vi "PWM Driver.vi"(5 "PWM Configuration (\"\")":string, 6 "Drv Refnum":T1, 7 "PWM Command":T2=enum."MEASURE", 8 "error in (no error)":errorcluster, 10 "PWM Stimulus":T4={"Zero"=FALSE, "Blank Screen"=FALSE, "Offset"=FALSE, "Offset Value"=4.0, "Frequency (MHz)"=0.0}) -> (0 "error out":errorcluster, 1 "Variant Output":string, 2 "PWM Measurement":T3 caption="This reading is always in the base units\ni.e. V, A, Ohms, Hz, Sec, etc." format="%#_10f", 4 "dup Drv Refnum":T1)   [LabVIEW 2011]
uses:
  PWM Measurement.ctl
  PWM Parameters.ctl
  PWM Command.ctl
  PWM Driver Ref.ctl
panel:
  in  "DEBUG?":bool
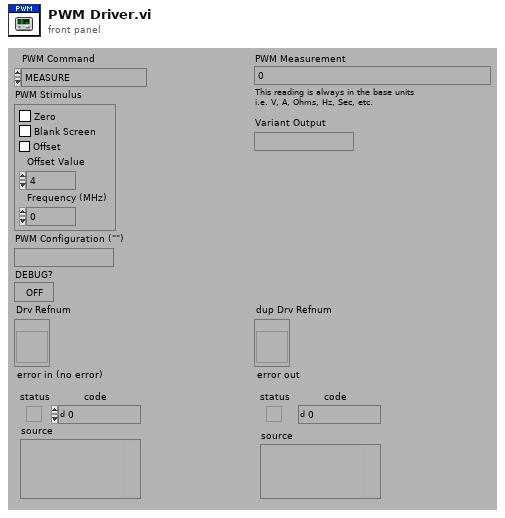
[diagram p1: front panel]
types:
  T1 = typedef "PWM Driver Ref.ctl" = refnum<vi>
  T2 = typedef "PWM Command.ctl" = enum16{"LOAD", "INITIALIZE", "PRESET", "GET STIMULUS", "SET STIMULUS", "MEASURE", "RELEASE", "UNLOAD", "GET CALIBRATION", "CALIBRATE"}
  T3 = typedef "PWM Measurement.ctl" = dbl
  T4 = typedef "PWM Parameters.ctl" = cluster{"Zero":bool, "Blank Screen":bool, "Offset":bool, "Offset Value":dbl, "Frequency (MHz)":dbl}
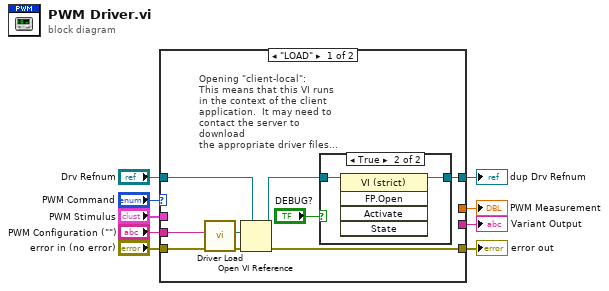
[diagram p0: block diagram]
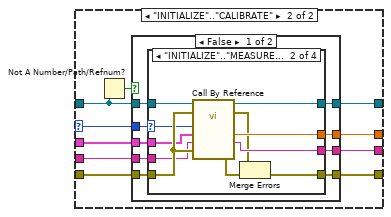
[diagram p3: hidden frame]
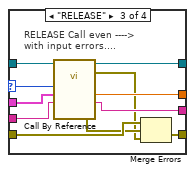
[diagram p5: hidden frame]
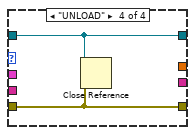
[diagram p6: hidden frame]
diagram:
  n1 = case shown="\"LOAD\"" "PWM Command" {
    selector: "PWM Command" -> [_ w24]
    tunnel: "error in (no error)" -> [w18 w31]
    tunnel: "PWM Stimulus" -> [_ w30]
    tunnel: [_ w29] -> w7
    tunnel: [w17 w28] -> w6
    tunnel: "PWM Configuration (\"\")" -> [w16 w27]
    tunnel: [_ w26] -> w4
    tunnel: [w15 w25] -> w3
    tunnel: "Drv Refnum" -> [w14 w23]
    frame "LOAD" {
      # "Opening \"client-local\":\nThis means that this VI runs\nin the context of the client\napplication.  It may need to\ncontact the server to download\nthe appropriate driver files..."
      n2 = call "Driver Load.vi"("error in (no error)"=w18, "DriverID DriverType (\"\")"=w16) -> ("error out"=w10:errorcluster, "Driver Component Path"=w11:path)  [unwired: 1 in, 7 out]
      n3 = Open VI Reference(type specifier VI Refnum (for type only)=w14, vi path=w11, error in (no error)=w10) -> (vi reference=w13:T1, error out=w17:errorcluster)  [unwired: 3 out]
      n4 = case shown="True" "DEBUG?" {
        tunnel: w13 -> [w19 w21]
        tunnel: [w19 w20] -> w15
        frame False {
        }
        frame True {
          n5 = invoke class="VI (strict)" method="FP.Open"(reference=w21) -> (reference out=w20:T1)  [unwired: 4 in, 4 out]
        }
      }
    }
    frame "INITIALIZE".."CALIBRATE" {
      n6 = Not A Number/Path/Refnum?(number/path/refnum=w23) -> (NaN/Path/Refnum?=w22:bool)
      n7 = case shown="False" w22 {
        tunnel: w31 -> [w40 w67]
        tunnel: w30 -> [w39 _]
        tunnel: [w38 _] -> w29
        tunnel: [w37 w67] -> w28
        tunnel: w27 -> [w36 _]
        tunnel: [w35 _] -> w26
        tunnel: [w34 w68] -> w25
        tunnel: w23 -> [w33 w68]
        tunnel: w24 -> [w32 _]
        frame False {
          n8 = case shown="\"INITIALIZE\"..\"MEASURE\", \"GET CALIBRATION\", \"CALIBRATE\"" w32 {
            selector: w32 -> [_ w45 w59 _]
            tunnel: w40 -> [w42 w46 w57 w65]
            tunnel: w39 -> [_ w43 w60 _]
            tunnel: [_ w50 w62 _] -> w38
            tunnel: [w42 w53 w64 w65] -> w37
            tunnel: w36 -> [_ w44 w58 _]
            tunnel: [_ w49 w61 _] -> w35
            tunnel: [w41 w51 w63 w66] -> w34
            tunnel: w33 -> [w41 w52 w54 w66]
            frame "LOAD", Default {
              # "This will not ever run."
            }
            frame "INITIALIZE".."MEASURE", "GET CALIBRATION", "CALIBRATE" {
              n9 = call-by-ref "?"(reference=w52, error in=w46, "error in (no error)"=w46, "PWM Configuration (\"\")"=w44, "PWM Stimulus"=w43, "PWM Command"=w45) -> (reference out=w51:T1, error out=w48:errorcluster, 0:"error out"=w47:errorcluster, "Variant Output"=w49:string, "PWM Measurement"=w50:T3)  [unwired: 5 in]
              n10 = Merge Errors(w48, w47) -> (w53:errorcluster)
            }
            frame "RELEASE" {
              # "RELEASE Call even ---->\nwith input errors...."
              n11 = call-by-ref "?"(reference=w54, "PWM Configuration (\"\")"=w58, "PWM Stimulus"=w60, "PWM Command"=w59) -> (reference out=w63:T1, error out=w55:errorcluster, 0:"error out"=w56:errorcluster, "Variant Output"=w61:string, "PWM Measurement"=w62:T3)  [unwired: 7 in]
              n12 = Merge Errors(w57, w56, w55) -> (w64:errorcluster)
            }
            frame "UNLOAD" {
              n13 = Close Reference(reference=w66, error in (no error)=w65) -> ()  [unwired: 1 out]
            }
          }
        }
        frame True {
          # "If the reference is not valid\nno operation is performed."
        }
      }
    }
  }
  "error out" <- w6
  "PWM Measurement" <- w7
  "Variant Output" <- w4
  "dup Drv Refnum" <- w3
